vi "Discret stage.vi"(0 "State":u32, 5 "N_curr":u32, 7 "N_stage":u32, 9 "Mode":u32) -> (4 "Preset_state":u32, 6 "St_on":bool, 8 "St_not_ok":bool, 10 "Curr_st_not_ok":bool)   [LabVIEW 2019]
uses:
  Logik/fronts.vi
  Trigers/RS.vi
  Timer Delay/Timers.lvlib
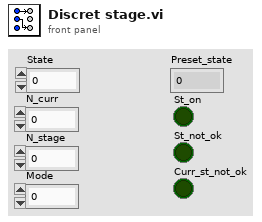
[diagram p1: front panel]
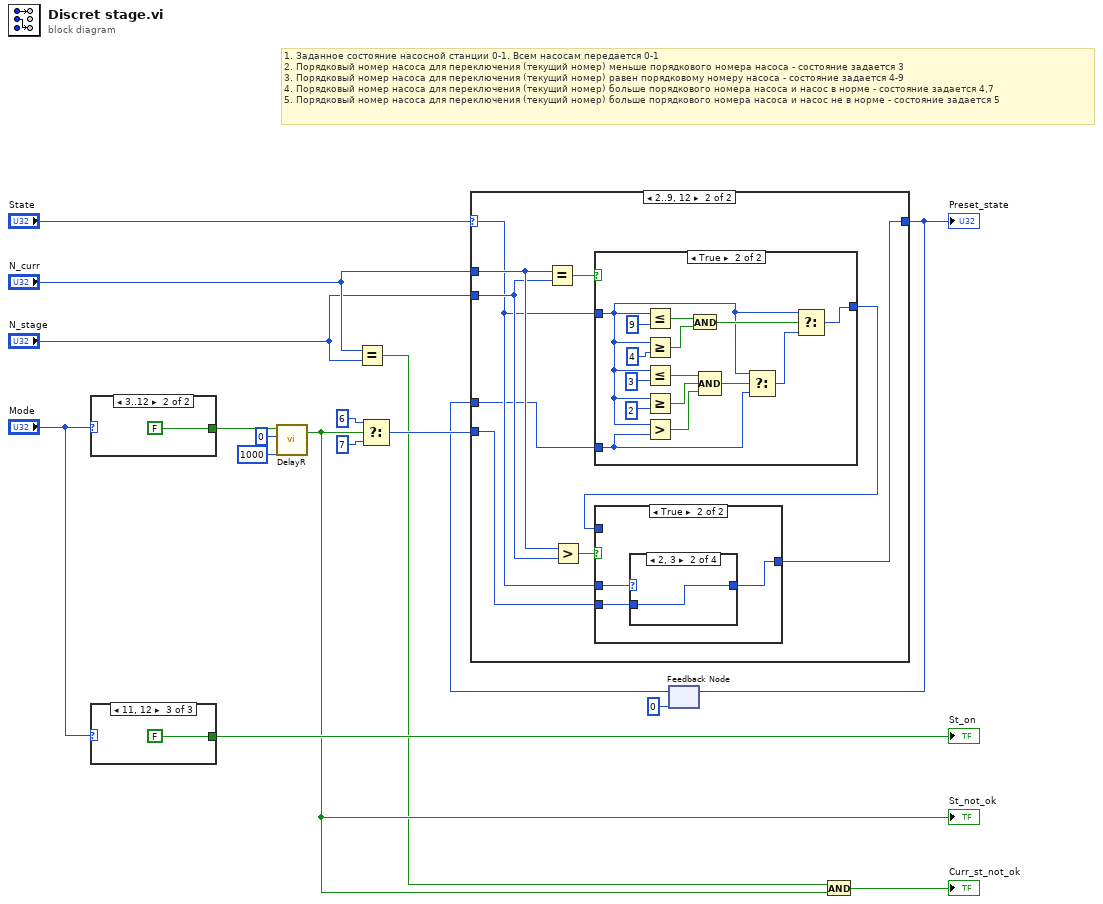
[diagram p0: block diagram]
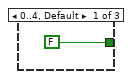
[diagram p2: hidden frame]
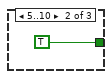
[diagram p3: hidden frame]
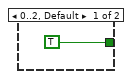
[diagram p4: hidden frame]
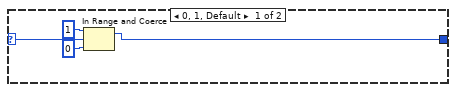
[diagram p5: hidden frame]
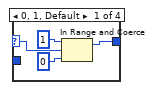
[diagram p7: hidden frame]
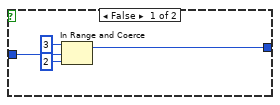
[diagram p10: hidden frame]
diagram:
  # "1. Заданное состояние насосной станции 0-1. Всем насосам передается 0-1\n2. Порядковый номер насоса для переключения (текущий номер) меньше порядкового номера насоса - состояние задается 3\n3. Порядковый номер насоса для переключения (текущий номер) равен порядковому номеру насоса - состояние задается 4-9\n4. Порядковый номер насоса для переключения (текущий номер) больше порядкового номера насоса и насос в норме - состояние задается 4,7\n5. Порядковый номер насоса для переключения (текущий номер) больше порядкового номера насоса и насос не в норме - состояние задается 5"
  n1 = case shown="3..12" "Mode" {
    tunnel: [TRUE FALSE] -> w16
    frame 0..2, Default {
    }
    frame 3..12 {
    }
  }
  n2 = case shown="11, 12" "Mode" {
    tunnel: [FALSE TRUE FALSE] -> w9
    frame 0..4, Default {
    }
    frame 5..10 {
    }
    frame 11, 12 {
    }
  }
  "St_on" <- w9
  n3 = call "DelayR.vi"("DelayOff"=u32 1000, "DelayOn"=u32 0, "In"=w16) -> ("Out"=w5:bool)  [unwired: 1 in, 1 out]
  "St_not_ok" <- w5
  n4 = Equal?(x="N_curr", y="N_stage") -> (x = y?=w4:bool)
  n5 = Select(t=u32 6, s=w5, f=u32 7) -> (s? t:f=w11:u32)
  n6 = feedback #1(u32 0 ("upper limit")) -> (w1:u32)
  n7 = case shown="2..9, 12" "State" {
    selector: "State" -> [w24 w31]
    tunnel: [w23 w28] -> w2
    tunnel: "N_curr" -> [_ w33]
    tunnel: "N_stage" -> [_ w32]
    tunnel: w11 -> [_ w30]
    tunnel: w1 -> [_ w27]
    frame 0, 1, Default {
      n8 = In Range and Coerce(upper limit=u32 1, x=w24, lower limit=u32 0) -> (coerced(x)=w23:u32)  [unwired: 1 out]
    }
    frame 2..9, 12 {
      n9 = Equal?(x=w33, y=w32) -> (x = y?=w35:bool)
      n10 = Greater?(x=w33, y=w32) -> (0:w34:bool)
      n11 = case shown="True" w35 {
        tunnel: w31 -> [w50 w51]
        tunnel: [w47 w65] -> w29
        tunnel: w27 -> [_ w62]
        frame False {
          n12 = In Range and Coerce(upper limit=u32 3, x=w50, lower limit=u32 2) -> (coerced(x)=w47:u32)  [unwired: 1 out]
        }
        frame True {
          n13 = Less Or Equal?(x=w51, y=u32 9 ("upper limit")) -> (x <= y?=w58:bool)
          n14 = Greater Or Equal?(x=w51, y=u32 4 ("lower limit")) -> (x >= y?=w57:bool)
          n15 = Less Or Equal?(x=w51, y=u32 3 ("upper limit")) -> (x <= y?=w52:bool)
          n16 = Greater Or Equal?(x=w51, y=u32 2 ("lower limit")) -> (x >= y?=w53:bool)
          n17 = Greater?(x=w51, y=w62) -> (0:w64:bool)
          n18 = And(x=w58, y=w57) -> (x .and. y?=w56:bool)
          n19 = Compound Arithmetic op=AND(w52, w53, w64) -> (w63:bool)
          n20 = Select(t=w51, s=w63, f=w62) -> (s? t:f=w61:u32)
          n21 = Select(t=w51, s=w56, f=w61) -> (s? t:f=w65:u32)
        }
      }
      n22 = case shown="True" w34 {
        tunnel: w29 -> [w36 _]
        tunnel: [w36 w37] -> w28
        tunnel: w31 -> [_ w39]
        tunnel: w30 -> [_ w38]
        frame False {
        }
        frame True {
          n23 = case shown="2, 3" w39 {
            selector: w39 -> [w41 _ w45 _]
            tunnel: [w40 w44 w45 w46] -> w37
            tunnel: w38 -> [_ w44 _ w46]
            frame 0, 1, Default {
              n24 = In Range and Coerce(upper limit=u8 1, x=w41, lower limit=u8 0) -> (coerced(x)=w40:u32)  [unwired: 1 out]
            }
            frame 2, 3 {
            }
            frame 4 {
            }
            frame 5..8 {
            }
          }
        }
      }
    }
  }
  "Preset_state" <- w2
  n25 = feedback-in #1(w2) -> ()
  n26 = And(x=w4, y=w5) -> (x .and. y?=→"Curr_st_not_ok":bool)
